vi "Main.vi"() -> ()   [LabVIEW 2017]
doc: "The myRIO Project template acquires acceleration data from the onboard accelerometer and displays the changes of acceleration values in a waveform chart."
uses:
  <vilib>/myRIO/Common/Instrument Driver Framework/myRIO v1.0/Encoder/typedefs/Encoder Count Direction Enum.ctl
  Motor Status Enum.ctl
  <vilib>/myRIO/Instrument Drivers/Onboard IO/PWM/typedefs/PWM Reference.ctl
  <vilib>/myRIO/Common/Instrument Driver Framework/Utilities/typedefs/myRIO Generic Hardware Reference.ctl
  <vilib>/myRIO/Common/Instrument Driver Framework/Utilities/typedefs/Hardware Version Enum.ctl
  <vilib>/myRIO/Common/Instrument Driver Framework/Utilities/typedefs/myRIO v1.0 Reference.ctl
  <vilib>/myRIO/Common/Instrument Driver Framework/Utilities/typedefs/Generic FPGA Reference.ctl
  <vilib>/myRIO/Common/Instrument Driver Framework/myRIO v1.0/PWM/typedefs/PWM Channels Enum.ctl
  <vilib>/myRIO/Instrument Drivers/Onboard IO/PWM/typedefs/PWM Configuration.ctl
  <vilib>/userdefined/High Color/nirio_resource_hc.ctl
  <vilib>/myRIO/Common/Instrument Driver Framework/Utilities/vis/Is FPGA Ref Available.vi
  <vilib>/myRIO/Common/Instrument Driver Framework/myRIO v1.0/PWM/vis/myRIO v1.1 Open PWM.vi
  <vilib>/myRIO/Instrument Drivers/Onboard IO/PWM/vis/Set Duty Cycle and Frequency.vi
  <vilib>/myRIO/Common/Instrument Driver Framework/Utilities/vis/Validate Channels.vi
  <vilib>/myRIO/Common/Instrument Driver Framework/myRIO v1.0/PWM/vis/myRIO v1.0 Reserve PWM.vi
  <vilib>/myRIO/Common/Instrument Driver Framework/myRIO v1.0/UART/vis/myRIO v1.0 Close UART.vi
  <vilib>/myRIO/Common/Instrument Driver Framework/myRIO v1.0/PWM/vis/myRIO v1.0 Build MUX Configuration PWM.vi
  <vilib>/myRIO/Common/Instrument Driver Framework/myRIO v1.0/Resource Manager/vis/myRIO v1.0 Reserve Channel List.vi
  <vilib>/myRIO/Common/Instrument Driver Framework/myRIO v1.0/Resource Manager/vis/myRIO v1.0 Create Configuration List.vi
  <vilib>/myRIO/Common/Instrument Driver Framework/myRIO v1.0/Resource Manager/vis/myRIO v1.0 Reserve Channel.vi
  <vilib>/myRIO/Common/Instrument Driver Framework/myRIO v1.0/Resource Manager/vis/myRIO v1.0 Unreserve Channel.vi
  <vilib>/myRIO/Common/Instrument Driver Framework/myRIO v1.0/Resource Manager/vis/myRIO v1.0 Build Mutex Name.vi
  <vilib>/Utility/VariantDataType/GetNumericInfo.vi
  <vilib>/Utility/error.llb/Error Cluster From Error Code.vi
  <vilib>/myRIO/Common/Instrument Driver Framework/myRIO v1.0/myRIO v1.1 Open.vi
  <vilib>/myRIO/Common/Instrument Driver Framework/Utilities/vis/IO Manager.vi
  <vilib>/myRIO/Common/Instrument Driver Framework/Utilities/vis/Configuration Manager.vi
  <vilib>/myRIO/Common/Instrument Driver Framework/myRIO v1.0/Resource Manager/vis/myRIO v1.0 Configure IO.vi
  <vilib>/myRIO/Common/Instrument Driver Framework/myRIO v1.0/myRIO v1.0 Close.vi
  <vilib>/myRIO/Common/Instrument Driver Framework/myRIO v1.0/PWM/vis/myRIO v1.0 Write PWM.vi
  <vilib>/myRIO/Common/Instrument Driver Framework/Utilities/vis/FPGA Ref Manager.vi
  <vilib>/myRIO/Common/Instrument Driver Framework/myRIO v1.0/myRIO v1.0 Reset FPGA.vi
  <vilib>/myRIO/Common/Instrument Driver Framework/myRIO v1.0/IRQ/vis/myRIO v1.0 IRQ Info FGV.vi
  <vilib>/myRIO/Common/Instrument Driver Framework/myRIO v1.0/IRQ/vis/myRIO v1.0 Timer IRQ Info FGV.vi
  <vilib>/myRIO/Common/Instrument Driver Framework/myRIO v1.0/IRQ/vis/myRIO v1.0 ISR Agent.vi
  <vilib>/myRIO/Express VI/Onboard IO/PWM/PWM Express VI.xnode
  <vilib>/myRIO/Instrument Drivers/Onboard IO/PWM/vis/myRIO PWM Open.xnode
  <vilib>/myRIO/Instrument Drivers/Utilities/Utilities.lvlib
  <vilib>/myRIO/Instrument Drivers/Onboard IO/PWM/PWM.lvlib
panel:
  in  "X Axis Motor Target":T1
  out "X Axis Motor Params":T2
  in  "Y Axis Motor Target":T3
  out "Y Axis Motor Params":T3
  in  "stop":bool
  out "Output String":string
  out "Encoder Output":T5
  out "Loop Iteration":i32
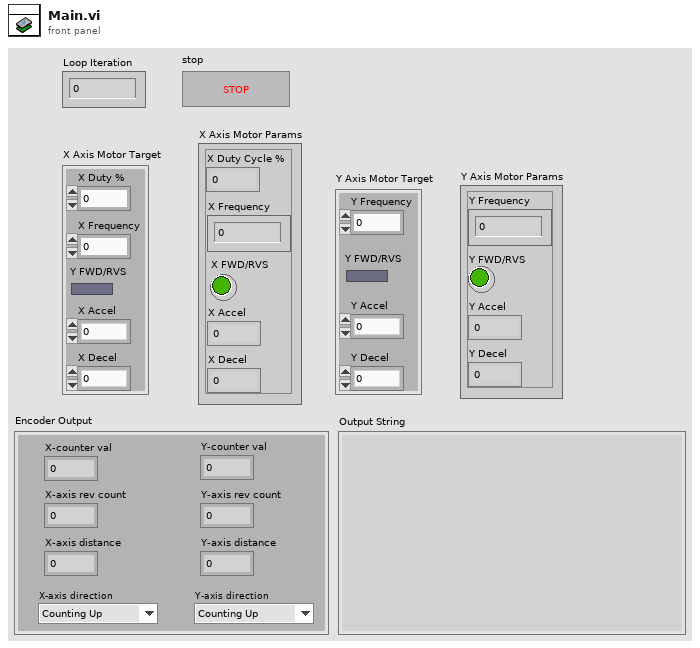
[diagram p1: front panel]
types:
  T1 = cluster{"X Frequency":dbl, "Y FWD/RVS":bool, "X Accel":dbl, "X Decel":dbl, "X Duty %":dbl}
  T2 = cluster{"X Frequency":dbl, "X FWD/RVS":bool, "X Accel":dbl, "X Decel":dbl, "X Duty Cycle %":dbl}
  T3 = cluster{"Y Frequency":dbl, "Y FWD/RVS":bool, "Y Accel":dbl, "Y Decel":dbl}
  T4 = typedef "Encoder Count Direction Enum.ctl" = enum16{"Counting Up", "Counting Down"}
  T5 = cluster{"Y-axis rev count":dbl, "Y-axis distance":dbl, "X-axis rev count":dbl, "X-axis distance":dbl, "Y-axis direction":T4, "X-axis direction":T4, "X-counter val":i32, "Y-counter val":i32}
  T6 = typedef "Motor Status Enum.ctl" = enum16{"Stop Motor", "Read Inputs", "Steady Speed", "Accelerate", "Decelerate"}
  T7 = cluster{dbl, "X-axis distance":dbl, "X Duty Cycle %":dbl, "X Frequency":dbl, "Y-axis distance":dbl, "Y Frequency":dbl, "X Accel":dbl, "X Decel":dbl, "Y Accel":dbl, "Y Decel":dbl}
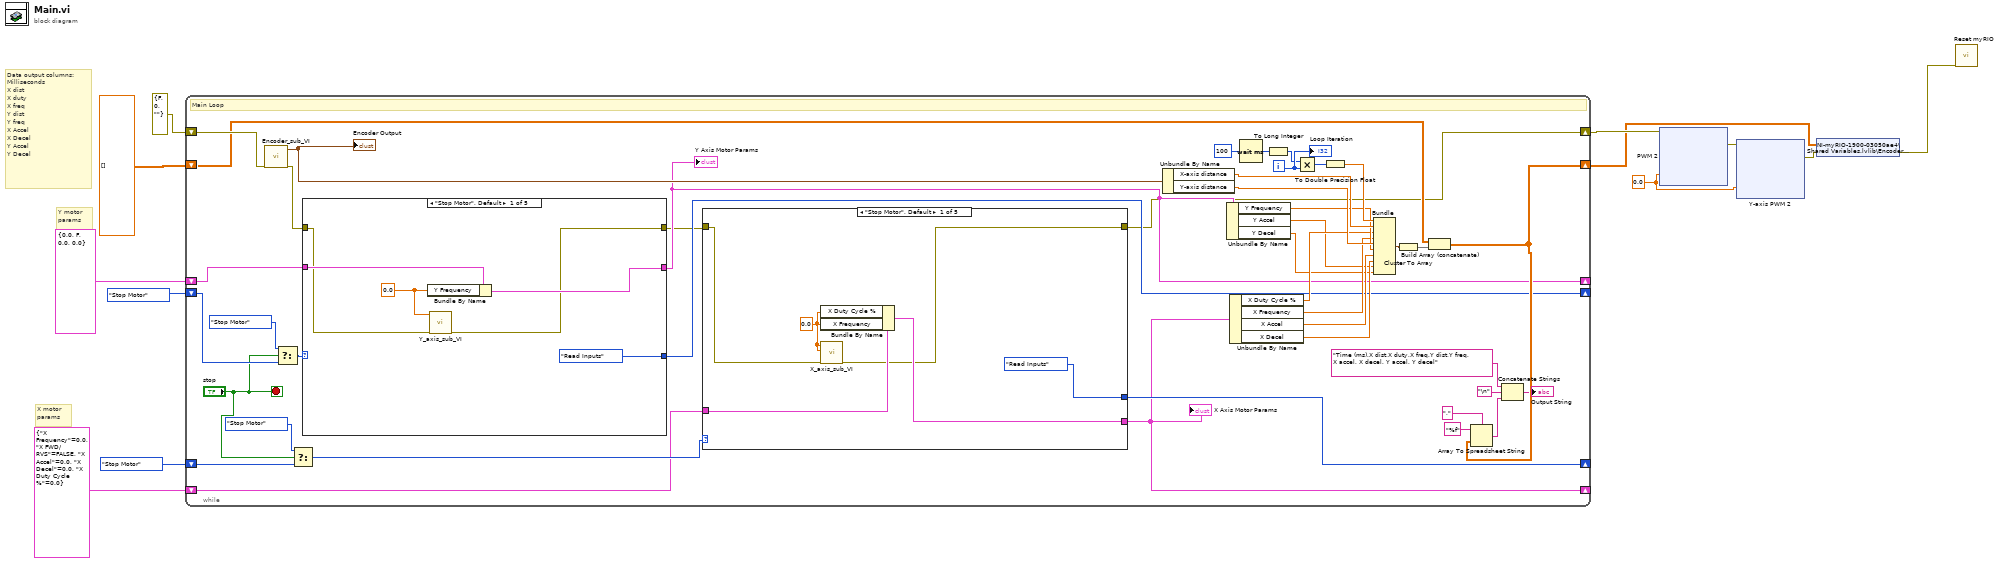
[diagram p0: block diagram]
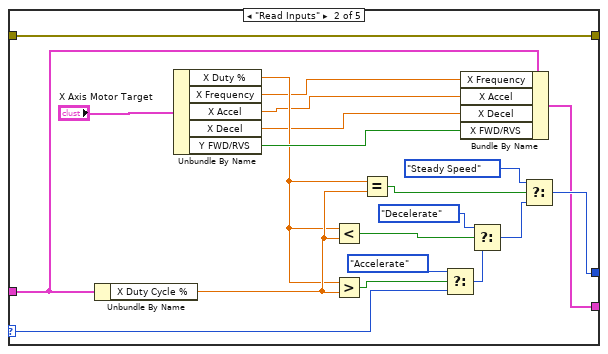
[diagram p2: hidden frame]
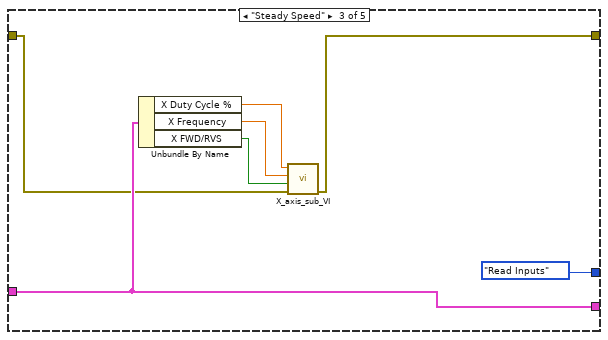
[diagram p3: hidden frame]
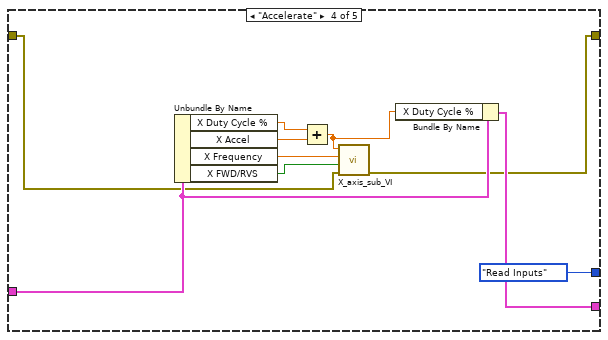
[diagram p4: hidden frame]
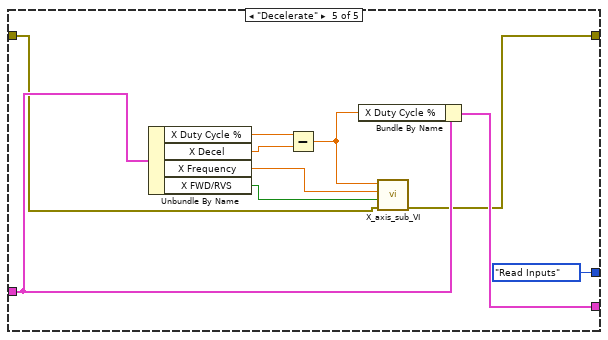
[diagram p5: hidden frame]
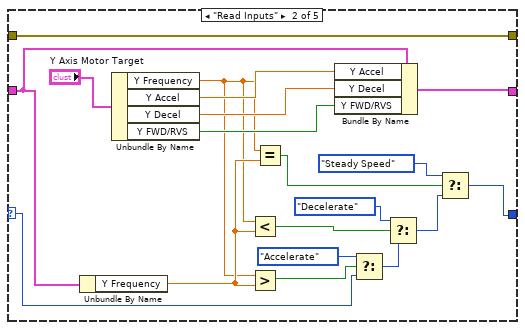
[diagram p6: hidden frame]
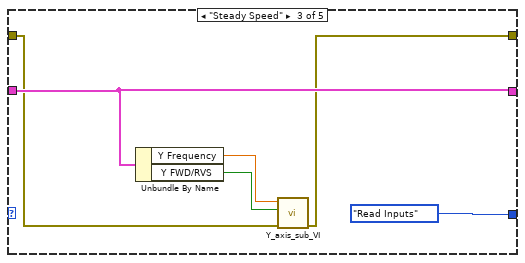
[diagram p7: hidden frame]
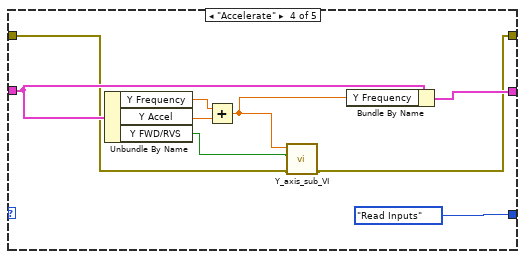
[diagram p8: hidden frame]
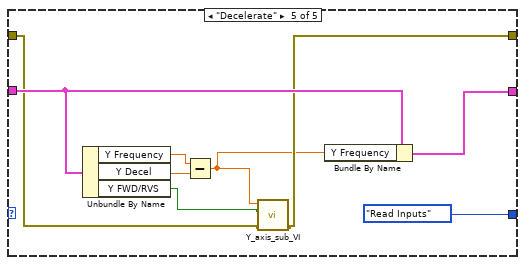
[diagram p9: hidden frame]
diagram:
  w5 = 0.0 ("Frequency [Hz]")
  # "X motor \nparams"
  # "Y motor \nparams"
  # "Data output columns:\nMilliseconds\nX dist\nX duty\nX freq\nY dist\nY freq\nX Accel\nX Decel\nY Accel\nY Decel"
  n1 = while {
    shift-right: [w20] -> w12
    shift-left: errorcluster {"status"=FALSE, "code"=0, "source"=""} ("error in (no error)") -> [w55]
    shift-right: [w50] -> w8
    shift-left: dbl[][] [] -> [w46]
    shift-right: [w29] -> _
    shift-left: T3 {"Y Frequency"=0.0, "Y FWD/RVS"=FALSE, "Y Accel"=0.0, "Y Decel"=0.0} ("Y Axis Motor Params 2") -> [w34]
    shift-right: [w33] -> _
    shift-left: Motor_Status_Enum."Stop Motor" -> [w31]
    shift-right: [w23] -> _
    shift-left: Motor_Status_Enum."Stop Motor" -> [w25]
    shift-right: [w19] -> _
    shift-left: T2 {"X Frequency"=0.0, "X FWD/RVS"=FALSE, "X Accel"=0.0, "X Decel"=0.0, "X Duty Cycle %"=0.0} ("X Axis Motor Params 3") -> [w22]
    i -> [w54]
    stop <- "stop" stop-if-true
    # "Main Loop"
    n2 = call "Encoder_sub_VI.vi"("error in (no error)"=w55) -> ("error out"=w28:errorcluster, "Encoder Output"=w53:T5)  [unwired: 9 in]
    "Encoder Output" <- w53
    n3 = Select(t=Motor_Status_Enum."Stop Motor", s="stop", f=w31) -> (s? t:f=w32:T6)
    n4 = Select(t=Motor_Status_Enum."Stop Motor", s="stop", f=w25) -> (s? t:f=w26:T6)
    n5 = case shown="\"Stop Motor\", Default" w32 {
      selector: w32 -> [_ w116 _ _ _]
      tunnel: w34 -> [w114 w118 w136 w145 w153]
      tunnel: [Motor_Status_Enum."Read Inputs" w117 Motor_Status_Enum."Read Inputs" Motor_Status_Enum."Read Inputs" Motor_Status_Enum."Read Inputs"] -> w33
      tunnel: [w112 w119 w136 w144 w154] -> w29
      tunnel: w28 -> [w110 w115 w135 w141 w151]
      tunnel: [w111 w115 w134 w140 w152] -> w21
      frame "Stop Motor", Default {
        w109 = 0.0 ("Y Frequency")
        n6 = Bundle By Name(cluster=w114, "Y Frequency"=w109) -> (w112:T3)
        n7 = call "Y_axis_sub_VI.vi"("error in (no error)"=w110, "Frequency"=w109) -> ("error out"=w111:errorcluster)  [unwired: 9 in]
      }
      frame "Read Inputs" {
        n8 = Unbundle By Name(w118) -> ("Y Frequency"=w126:dbl)
        n9 = Unbundle By Name("Y Axis Motor Target") -> ("Y Frequency"=w125:dbl, "Y Accel"=w130:dbl, "Y Decel"=w131:dbl, "Y FWD/RVS"=w132:bool)
        n10 = Less?(x=w125, y=w126) -> (x < y?=w122:bool)
        n11 = Greater?(x=w125, y=w126) -> (0:w133:bool)
        n12 = Equal?(x=w125, y=w126) -> (x = y?=w127:bool)
        n13 = Bundle By Name(cluster=w118, "Y Accel"=w130, "Y Decel"=w131, "Y FWD/RVS"=w132) -> (w119:T3)
        n14 = Select(t=Motor_Status_Enum."Accelerate", s=w133, f=w116) -> (s? t:f=w124:T6)
        n15 = Select(t=Motor_Status_Enum."Decelerate", s=w122, f=w124) -> (s? t:f=w128:T6)
        n16 = Select(t=Motor_Status_Enum."Steady Speed", s=w127, f=w128) -> (s? t:f=w117:T6)
      }
      frame "Steady Speed" {
        n17 = Unbundle By Name(w136) -> ("Y Frequency"=w138:dbl, "Y FWD/RVS"=w139:bool)
        n18 = call "Y_axis_sub_VI.vi"("error in (no error)"=w135, "FWD/RVS"=w139, "Frequency"=w138) -> ("error out"=w134:errorcluster)  [unwired: 8 in]
      }
      frame "Accelerate" {
        n19 = Unbundle By Name(w145) -> ("Y Frequency"=w147:dbl, "Y Accel"=w148:dbl, "Y FWD/RVS"=w142:bool)
        n20 = Add(x=w147, y=w148) -> (x+y=w143:dbl)
        n21 = call "Y_axis_sub_VI.vi"("error in (no error)"=w141, "FWD/RVS"=w142, "Frequency"=w143) -> ("error out"=w140:errorcluster)  [unwired: 8 in]
        n22 = Bundle By Name(cluster=w145, "Y Frequency"=w143) -> (w144:T3)
      }
      frame "Decelerate" {
        n23 = Unbundle By Name(w153) -> ("Y Frequency"=w157:dbl, "Y Decel"=w156:dbl, "Y FWD/RVS"=w150:bool)
        n24 = Subtract(x=w157, y=w156) -> (x-y=w149:dbl)
        n25 = call "Y_axis_sub_VI.vi"("error in (no error)"=w151, "FWD/RVS"=w150, "Frequency"=w149) -> ("error out"=w152:errorcluster)  [unwired: 8 in]
        n26 = Bundle By Name(cluster=w153, "Y Frequency"=w149) -> (w154:T3)
      }
    }
    "Y Axis Motor Params" <- w29
    n27 = case shown="\"Stop Motor\", Default" w26 {
      selector: w26 -> [_ w67 _ _ _]
      tunnel: [Motor_Status_Enum."Read Inputs" w66 Motor_Status_Enum."Read Inputs" Motor_Status_Enum."Read Inputs" Motor_Status_Enum."Read Inputs"] -> w23
      tunnel: [w58 w65 w85 w92 w102] -> w19
      tunnel: w22 -> [w59 w64 w85 w91 w101]
      tunnel: w21 -> [w57 w62 w83 w90 w100]
      tunnel: [w56 w62 w82 w89 w99] -> w20
      frame "Stop Motor", Default {
        w61 = 0.0 ("Y Frequency")
        n28 = Bundle By Name(cluster=w59, "X Duty Cycle %"=w61, "X Frequency"=w61) -> (w58:T2)
        n29 = call "X_axis_sub_VI.vi"("error in (no error)"=w57, "Frequency"=w61, "Duty Cycle %"=w61) -> ("error out"=w56:errorcluster)  [unwired: 8 in]
      }
      frame "Read Inputs" {
        n30 = Unbundle By Name(w64) -> ("X Duty Cycle %"=w79:dbl)
        n31 = Unbundle By Name("X Axis Motor Target") -> ("X Duty %"=w78:dbl, "X Frequency"=w70:dbl, "X Accel"=w68:dbl, "X Decel"=w69:dbl, "Y FWD/RVS"=w81:bool)
        n32 = Less?(x=w78, y=w79) -> (x < y?=w73:bool)
        n33 = Greater?(x=w78, y=w79) -> (0:w71:bool)
        n34 = Equal?(x=w78, y=w79) -> (x = y?=w77:bool)
        n35 = Select(t=Motor_Status_Enum."Accelerate", s=w71, f=w67) -> (s? t:f=w75:T6)
        n36 = Bundle By Name(cluster=w64, "X Frequency"=w70, "X Accel"=w68, "X Decel"=w69, "X FWD/RVS"=w81) -> (w65:T2)
        n37 = Select(t=Motor_Status_Enum."Decelerate", s=w73, f=w75) -> (s? t:f=w76:T6)
        n38 = Select(t=Motor_Status_Enum."Steady Speed", s=w77, f=w76) -> (s? t:f=w66:T6)
      }
      frame "Steady Speed" {
        n39 = Unbundle By Name(w85) -> ("X Duty Cycle %"=w87:dbl, "X Frequency"=w86:dbl, "X FWD/RVS"=w88:bool)
        n40 = call "X_axis_sub_VI.vi"("error in (no error)"=w83, "FWD/RVS"=w88, "Frequency"=w86, "Duty Cycle %"=w87) -> ("error out"=w82:errorcluster)  [unwired: 7 in]
      }
      frame "Accelerate" {
        n41 = Unbundle By Name(w91) -> ("X Duty Cycle %"=w94:dbl, "X Accel"=w95:dbl, "X Frequency"=w96:dbl, "X FWD/RVS"=w98:bool)
        n42 = Add(x=w94, y=w95) -> (x+y=w97:dbl)
        n43 = call "X_axis_sub_VI.vi"("error in (no error)"=w90, "FWD/RVS"=w98, "Frequency"=w96, "Duty Cycle %"=w97) -> ("error out"=w89:errorcluster)  [unwired: 7 in]
        n44 = Bundle By Name(cluster=w91, "X Duty Cycle %"=w97) -> (w92:T2)
      }
      frame "Decelerate" {
        n45 = Unbundle By Name(w101) -> ("X Duty Cycle %"=w104:dbl, "X Decel"=w105:dbl, "X Frequency"=w106:dbl, "X FWD/RVS"=w108:bool)
        n46 = Subtract(x=w104, y=w105) -> (x-y=w107:dbl)
        n47 = Bundle By Name(cluster=w101, "X Duty Cycle %"=w107) -> (w102:T2)
        n48 = call "X_axis_sub_VI.vi"("error in (no error)"=w100, "FWD/RVS"=w108, "Frequency"=w106, "Duty Cycle %"=w107) -> ("error out"=w99:errorcluster)  [unwired: 7 in]
      }
    }
    "X Axis Motor Params" <- w19
    n49 = Unbundle By Name(w53) -> ("X-axis distance"=w49:dbl, "Y-axis distance"=w48:dbl)
    n50 = Unbundle By Name(w29) -> ("Y Frequency"=w45:dbl, "Y Accel"=w40:dbl, "Y Decel"=w39:dbl)
    n51 = Unbundle By Name(w19) -> ("X Duty Cycle %"=w44:dbl, "X Frequency"=w43:dbl, "X Accel"=w42:dbl, "X Decel"=w41:dbl)
    n52 = Wait (ms)(milliseconds to wait=u32 100) -> (millisecond timer value=w35:u32)
    n53 = To Long Integer(number=w35) -> (32bit integer=w38:i32)
    n54 = Multiply(x=w38, y=w54) -> (x*y=w36:i32)
    n55 = To Double Precision Float(number=w36) -> (double precision float=w47:dbl)
    n56 = Bundle(w47, "X-axis distance"=w49, "X Duty Cycle %"=w44, "X Frequency"=w43, "Y-axis distance"=w48, "Y Frequency"=w45, "X Accel"=w42, "X Decel"=w41, "Y Accel"=w40, "Y Decel"=w39) -> (w51:T7)  [unwired: 1 in]
    n57 = Cluster To Array(cluster=w51) -> (array=w52:dbl[])
    n58 = Build Array (concatenate)(w46, w52) -> (w50:dbl[][])
    n59 = Array To Spreadsheet String(delimiter (Tab)=",", array=w50, 3:"%f" ("format string")) -> (spreadsheet string=w17:string)
    n60 = Concatenate Strings("Time (ms),X dist,X duty,X freq,Y dist,Y freq, X accel, X decel, Y accel, Y decel", "\n", w17) -> (→"Output String":string)
    "Loop Iteration" <- w54
  }
  n61 = xnode "PWM 2"("Frequency [Hz]"=w5, "error in (no error)"=w12) -> ("error out"=w7:errorcluster)
  n62 = xnode "Y-axis PWM 2"("Frequency [Hz]"=w5, "error in (no error)"=w7) -> ("error out"=w6:errorcluster)
  n63 = shared-variable "NI-myRIO-1900-03050ae4\\Shared Variables.lvlib\\Encoder Data"(w8, error in=w6) -> (error out=w9:errorcluster)
  n64 = call <vilib>:"Reset myRIO.vi"("error in (no error)"=w9) -> ()  [unwired: 10 in, 1 out]
